vi "Update Scalar Channel GUID.vi"(8 "error in (no error)":errorcluster, 10 "Data Type":T2 format="%.0x", 11 "item ref in":T1 format="%.0x") -> (0 "error out":errorcluster, 3 "item ref out":T1 format="%.0x")   [LabVIEW 2018, in "FPGA Addon System Explorer.lvlib"]
uses:
  FPGA Addon System Explorer.lvlib
  <vilib>/NI Veristand/Custom Device API/Custom Device Item Ref.ctl
  Addon Shared/Types/FPGA Addon Data Type.ctl
  Addon Shared/SubVIs/Constants.vi
  <vilib>/NI Veristand/Custom Device API/Custom Device API.lvlib
  Addon Shared/FPGA Addon Shared.lvlib
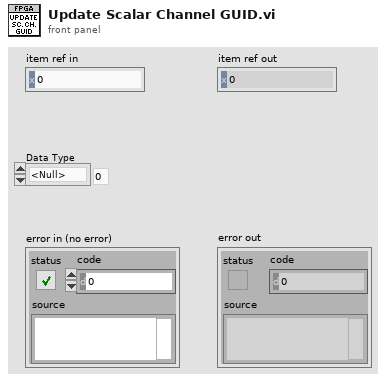
[diagram p1: front panel]
types:
  T1 = typedef "Custom Device API.lvlib/Custom Device Item Ref.ctl" = u64
  T2 = typedef "FPGA Addon Shared.lvlib/FPGA Addon Data Type.ctl" = enum8{"<Null>", "I8", "I16", "I32", "I64", "U8", "U16", "U32", "U64", "SGL", "Boolean", "Analog PWM In Settings", "Analog PWM In", "Digital PWM In Settings", "Digital PWM In", "Digital PWM Out", "Sine Out", "FXP", "FXP+/-24.5", "FXP+/-16.5", "FXP+/-32.8", "FXP+/-64.32", "FXP+/-16.7", "FXP+/-20.5", "FXP+/-27.5", "FXP+/-32.16", "FXP+16.3", "FXP+18.3", "Digital Static In", "Digital Static Out", "Digital Static In Settings", "Digital WSS Out", "Quad Encoder Settings", "Quad Encoder In", "Group"}
  T3 = typedef "Custom Device API.lvlib/Custom Device Item Info.ctl" = cluster{"Name":string, "Is Channel":bool, "GUID":string, "Is Waveform":bool}
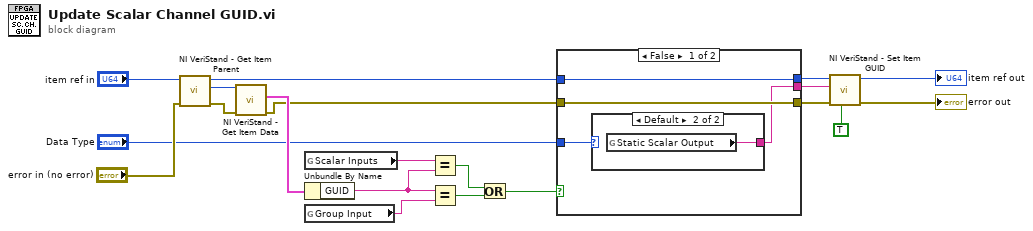
[diagram p0: block diagram]
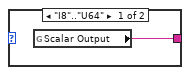
[diagram p2: hidden frame]
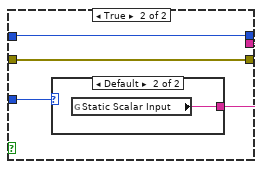
[diagram p3: hidden frame]
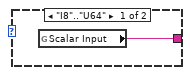
[diagram p4: hidden frame]
diagram:
  n1 = call <vilib>:"NI VeriStand - Get Item Parent.vi"("error in (no error)"="error in (no error)", "Item Ref in"="item ref in") -> ("error out"=w18:errorcluster, "Parent Ref"=w17:T1, "Item Ref out"=w7:T1)  [unwired: 6 in, 1 out]
  n2 = call <vilib>:"NI VeriStand - Get Item Data.vi"("error in (no error)"=w18, "Item Ref in"=w17) -> ("error out"=w8:errorcluster, "Item Info"=w16:T3)  [unwired: 6 in, 2 out]
  n3 = global read "Constants.vi" "Scalar Inputs"() -> (w13:string)
  n4 = Unbundle By Name(w16) -> ("GUID"=w12:string)
  n5 = global read "Constants.vi" "Group Input"() -> (w15:string)
  n6 = Equal?(x=w13, y=w12) -> (x = y?=w11:bool)
  n7 = Equal?(x=w12, y=w15) -> (x = y?=w14:bool)
  n8 = Or(x=w11, y=w14) -> (x .or. y?=w10:bool)
  n9 = case shown="False" w10 {
    tunnel: "Data Type" -> [w24 w30]
    tunnel: w8 -> [w22 w29]
    tunnel: w7 -> [w23 w27]
    tunnel: [w22 w29] -> w3
    tunnel: [w21 w28] -> w5
    tunnel: [w23 w27] -> w4
    frame False {
      n10 = case shown="Default" w24 {
        tunnel: [w25 w26] -> w21
        frame "I8".."U64" {
          n11 = global read "Constants.vi" "Scalar Output"() -> (w25:string)
        }
        frame Default {
          n12 = global read "Constants.vi" "Static Scalar Output"() -> (w26:string)
        }
      }
    }
    frame True {
      n13 = case shown="Default" w30 {
        tunnel: [w31 w32] -> w28
        frame "I8".."U64" {
          n14 = global read "Constants.vi" "Scalar Input"() -> (w31:string)
        }
        frame Default {
          n15 = global read "Constants.vi" "Static Scalar Input"() -> (w32:string)
        }
      }
    }
  }
  n16 = call <vilib>:"NI VeriStand - Set Item GUID.vi"("Refresh System Explorer Tree? (F)"=TRUE, "error in (no error)"=w3, "GUID"=w5, "Item Ref in"=w4) -> ("error out"=→"error out":errorcluster, "Item Ref out"=→"item ref out":T1)  [unwired: 6 in]
